vi "IVCurve Edit.vi"() -> ()   [LabVIEW 2019]
uses:
  Classes/Settings/Setting Database/Setting Database.lvclass
  Classes/Settings/Dot Settings/Dot Settings.lvclass
  Classes/Settings/Dot Settings/TypeDefs/IV Settings.ctl
  Classes/Settings/Dot Settings/Dot Settings.lvclass/Dot Settings.ctl
  <vilib>/JKI/JKI SMO/SMO/SMO.lvclass
panel:
  in  "Time":dbl caption="Time (s)"
  in  "Critical Points (V)":dbl[](array[numeric])
  out "Beta String":string
  in  "Pattern":T1(ring) caption="Enum"
  in  "Cycles":i32
  in  "Port":u32
  in  "End":dbl caption="End (V)"
  in  "Start":dbl caption="Start (V)"
  in  "Rate":dbl caption="Rate (V/s)"
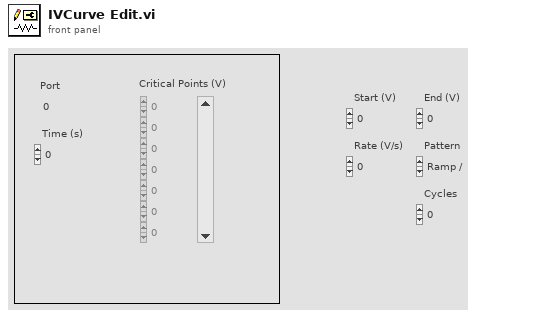
[diagram p1: front panel]
types:
  T1 = enum16{"Ramp /", "Ramp /\\", "Smooth Ramp _/", "Smooth Ramp _/\\_", "Frequency"}
  T2 = enum32{"Invalid", "Standard", "Closed", "Hidden", "Minimized", "Maximized"}
  T3 = enum32{"invalid app kind", "Development System", "Run Time System", "Student Edition", "Embedded LabVIEW", "Evaluation", "Custom"}
  T4 = typedef "Setting Database.lvclass/PublicEvents--Setting Database.NewActiveDot.ctl" = refnum<class "Dot Settings.lvclass">
  T5 = cluster{"Core":cluster{"Current VI Reference":refnum<vi>, "Close Panel on Exit?":bool}, "SettingDB":refnum<class "Setting Database.lvclass">, "Dot Settings":refnum<class "Dot Settings.lvclass">}
  T6 = typedef "Dot Settings.lvclass/IV Settings.ctl" = cluster{"Pattern":enum16{"Ramp /", "Ramp /\\", "Smooth Ramp _/", "Smooth Ramp _/\\_", "Frequency"}, "Cycles":i32, "Rate":dbl, "End":dbl, "Start":dbl, "Port":u32, "Time":dbl, "Points":dbl[]}
  T7 = cluster{"Current VI Reference":refnum<vi>, "Close Panel on Exit?":bool}
  T8 = typedef "Setting Database.lvclass/PublicEvents--Cluster.ctl" = cluster{"NewActivePath":refnum<user-event>, "PathsUpdated":refnum<user-event>, "RectanglesUpdated":refnum<user-event>, "NewActiveRectangle":refnum<user-event>, "NewActiveFunnel":refnum<user-event>, "FunnelsUpdated":refnum<user-event>, "NewActiveDot":refnum<user-event>, "DotsUpdated":refnum<user-event>}
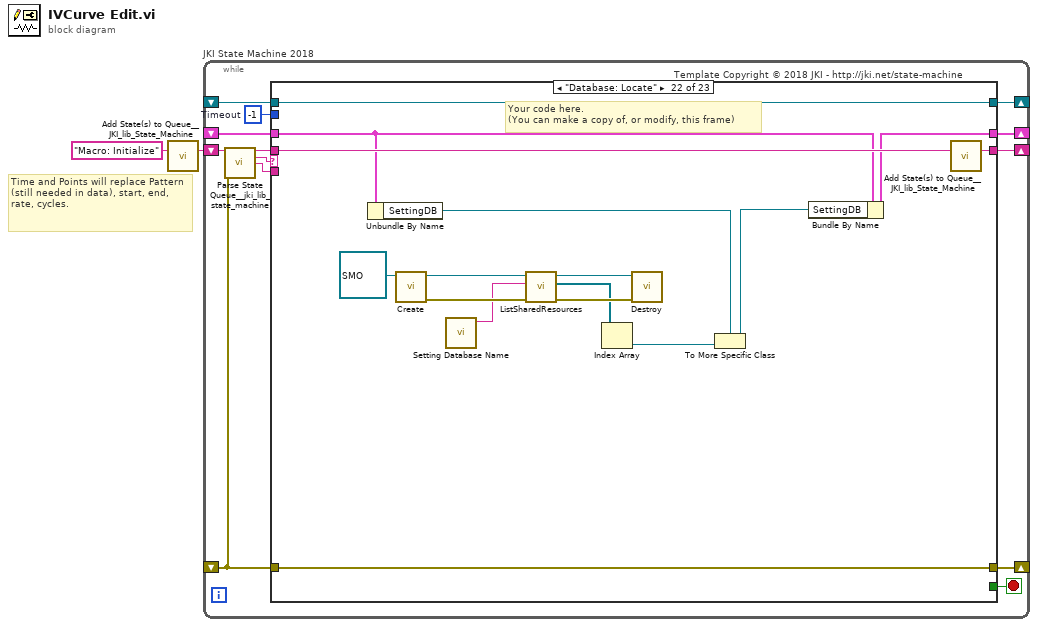
[diagram p0: block diagram]
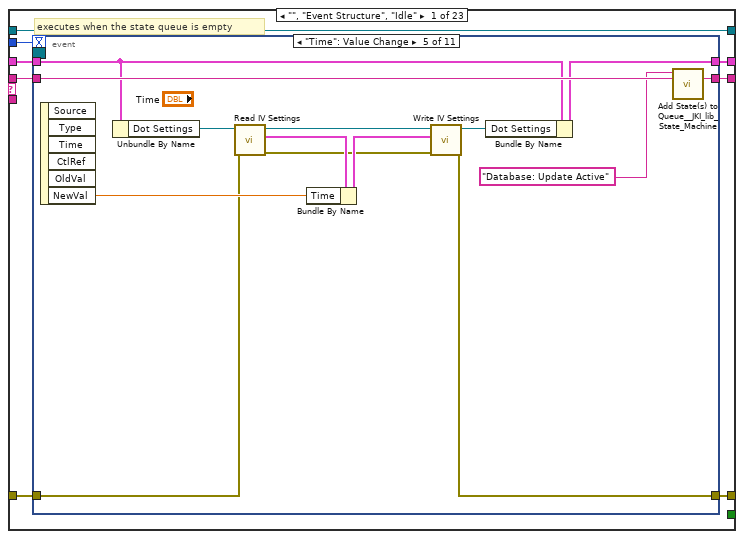
[diagram p2: hidden frame]
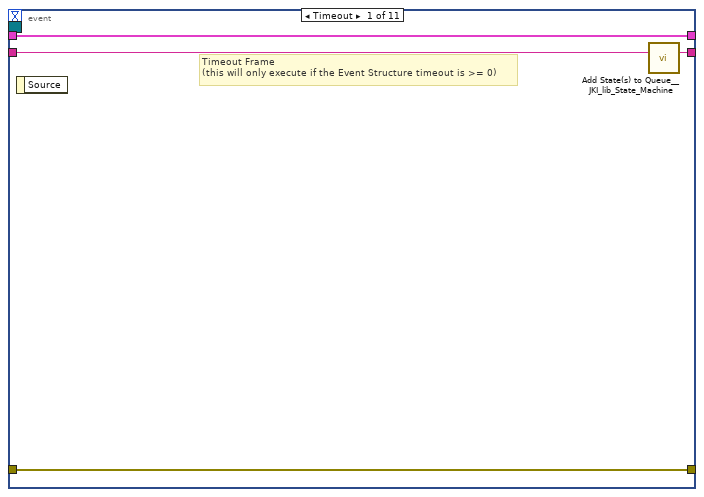
[diagram p3: hidden frame]
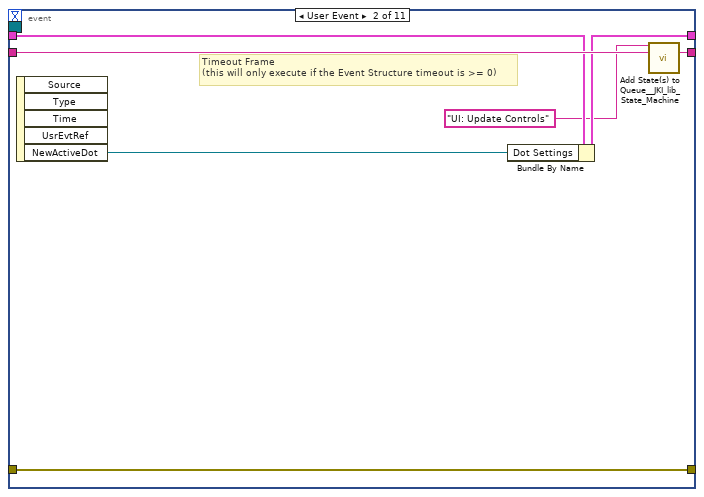
[diagram p4: hidden frame]
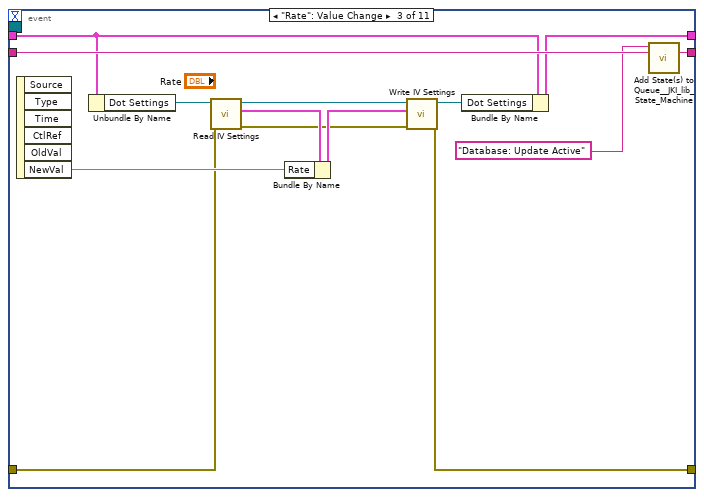
[diagram p5: hidden frame]
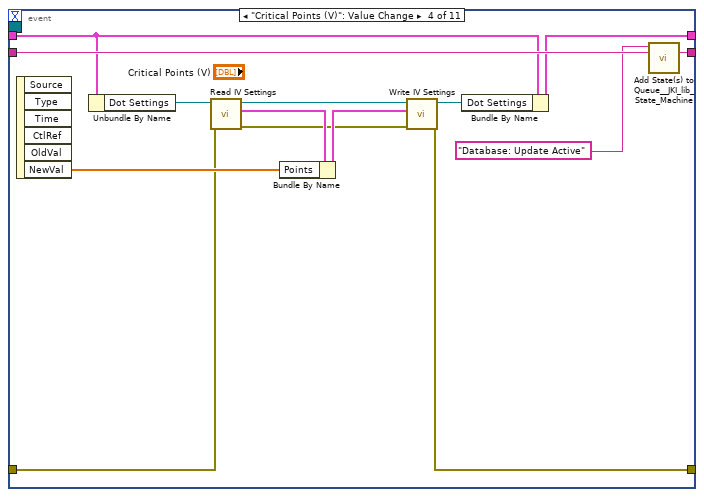
[diagram p6: hidden frame]
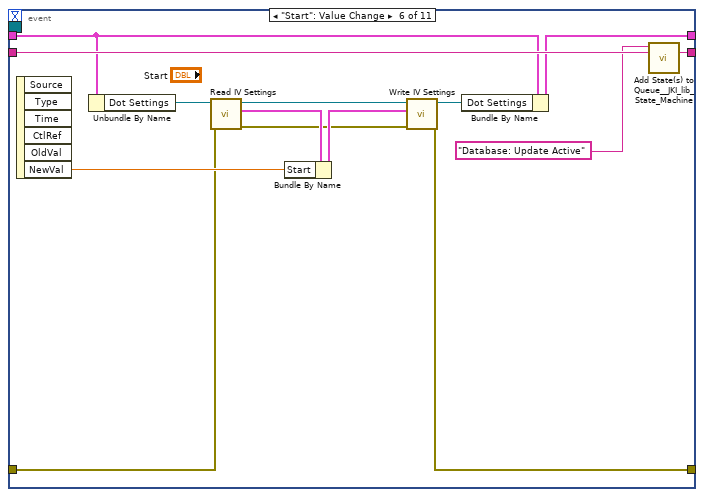
[diagram p7: hidden frame]
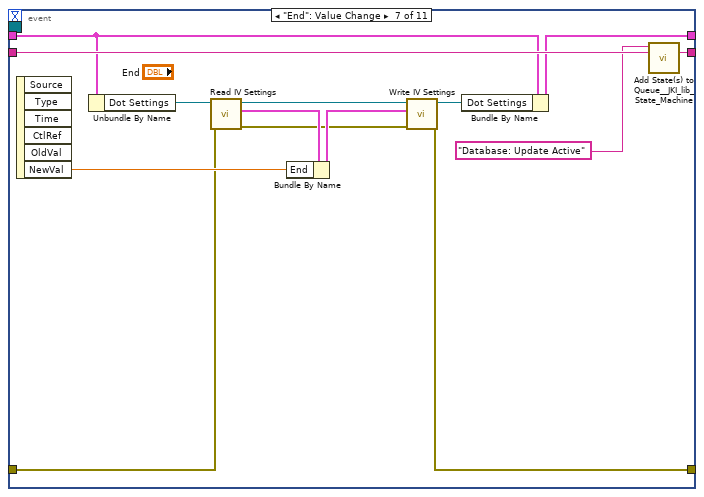
[diagram p8: hidden frame]
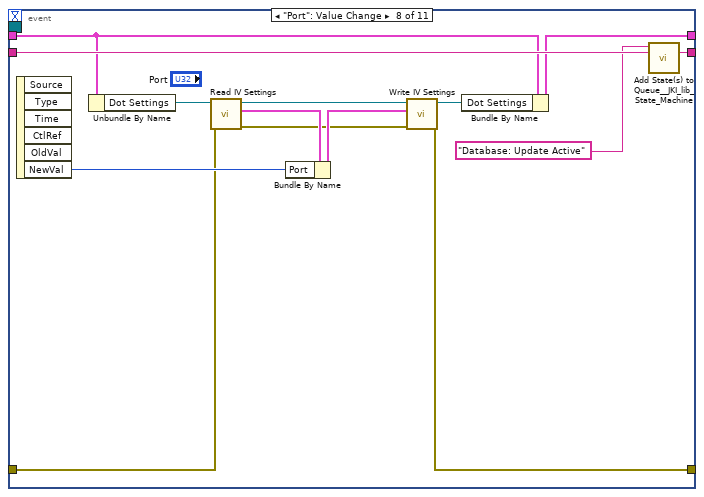
[diagram p9: hidden frame]
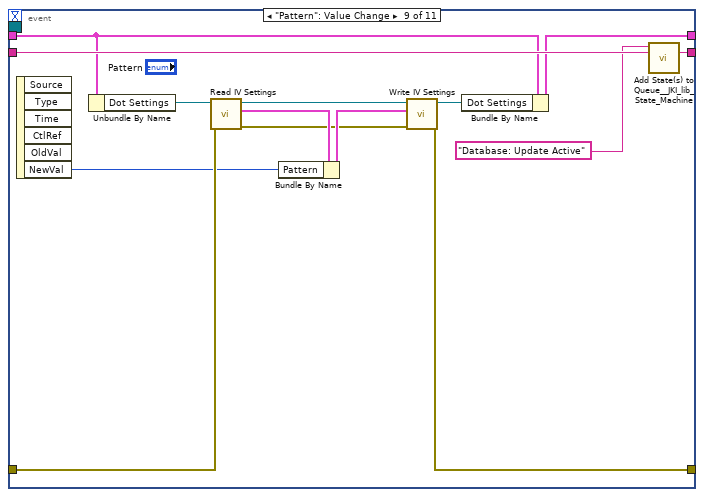
[diagram p10: hidden frame]
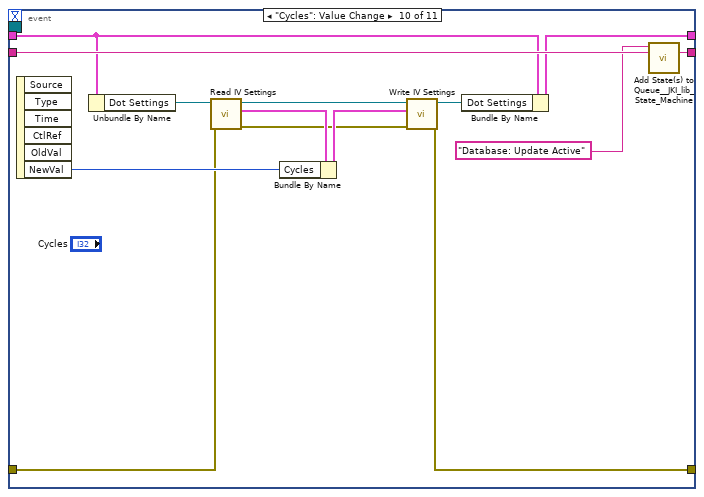
[diagram p11: hidden frame]
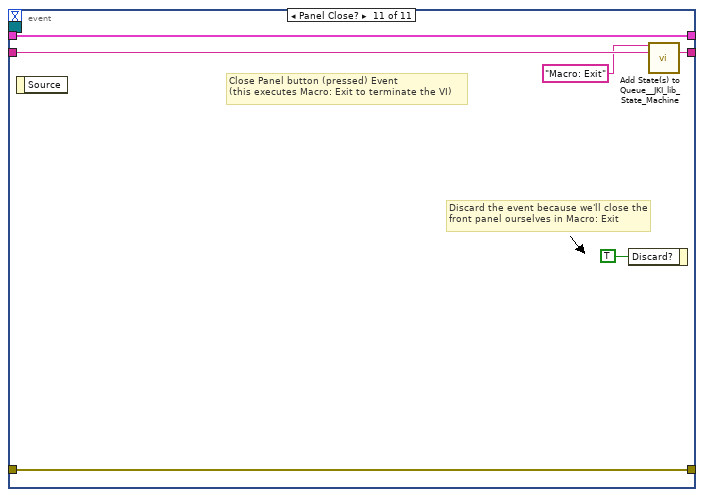
[diagram p12: hidden frame]
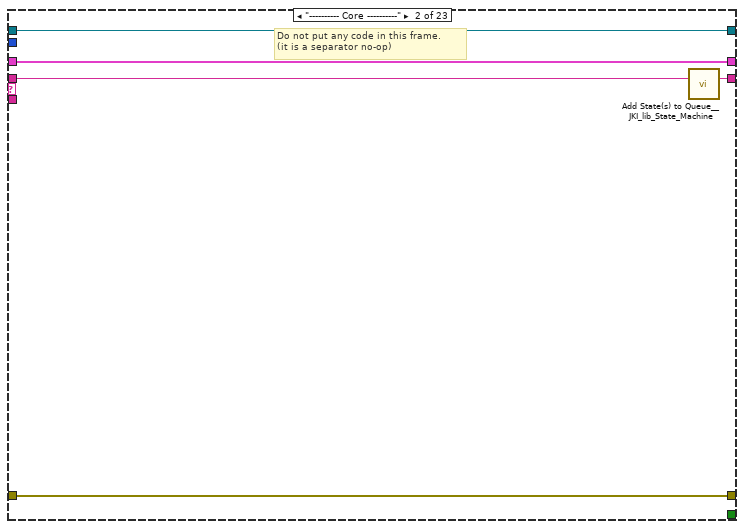
[diagram p13: hidden frame]
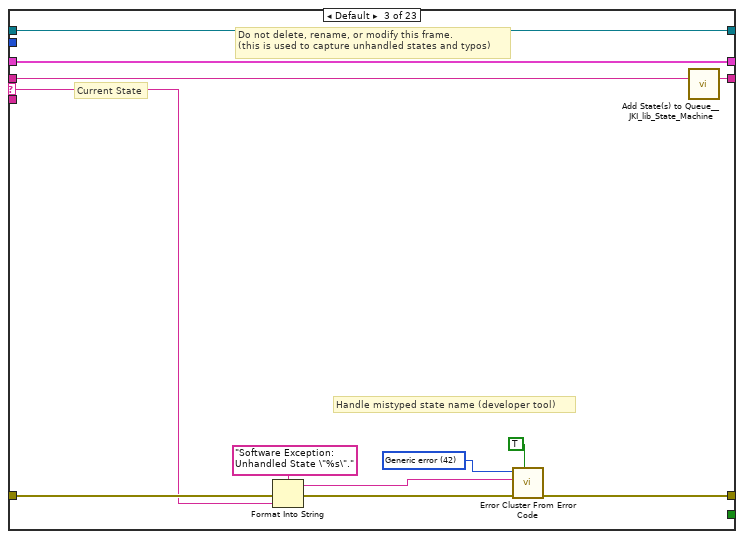
[diagram p14: hidden frame]
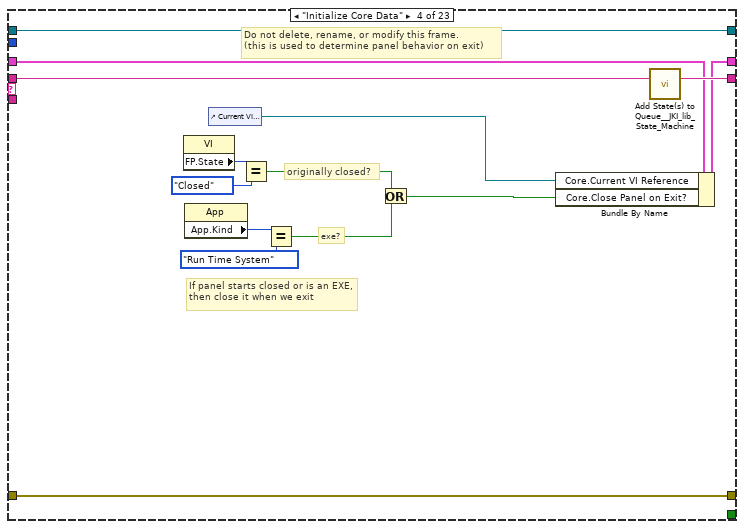
[diagram p15: hidden frame]
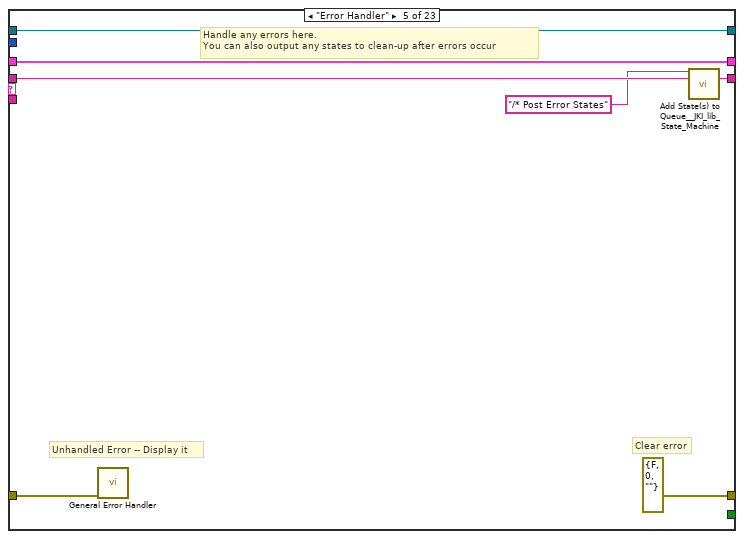
[diagram p16: hidden frame]
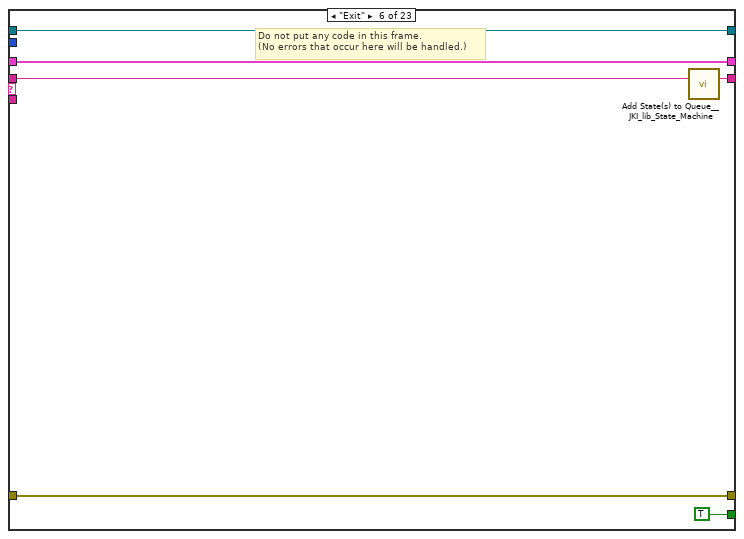
[diagram p17: hidden frame]
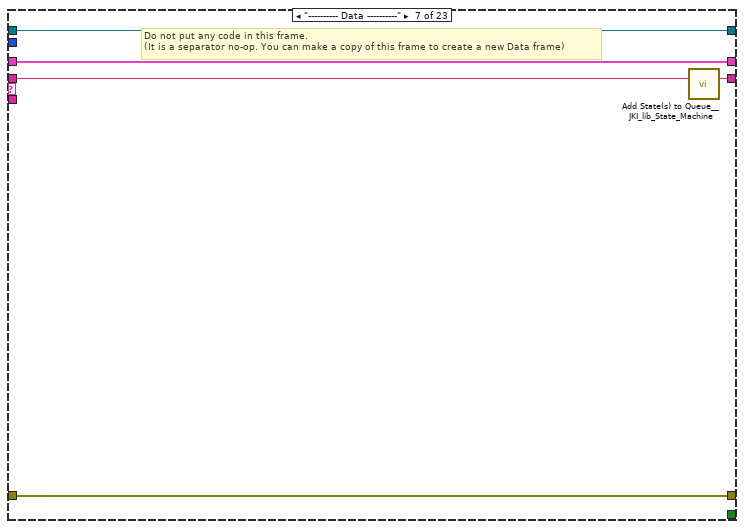
[diagram p18: hidden frame]
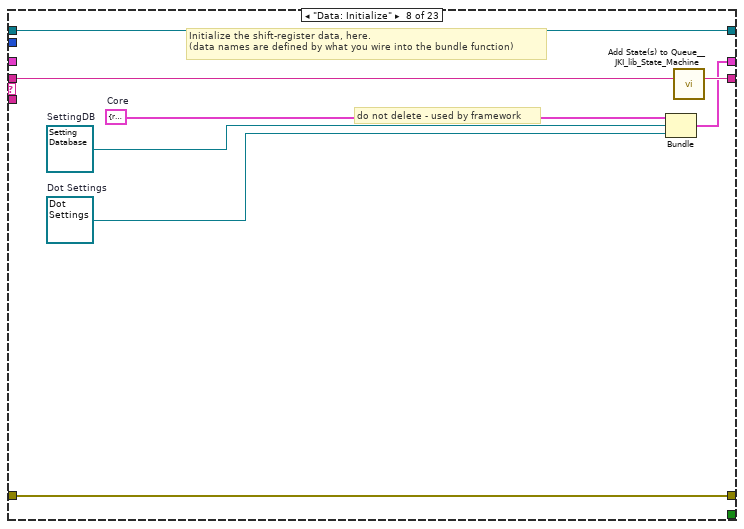
[diagram p19: hidden frame]
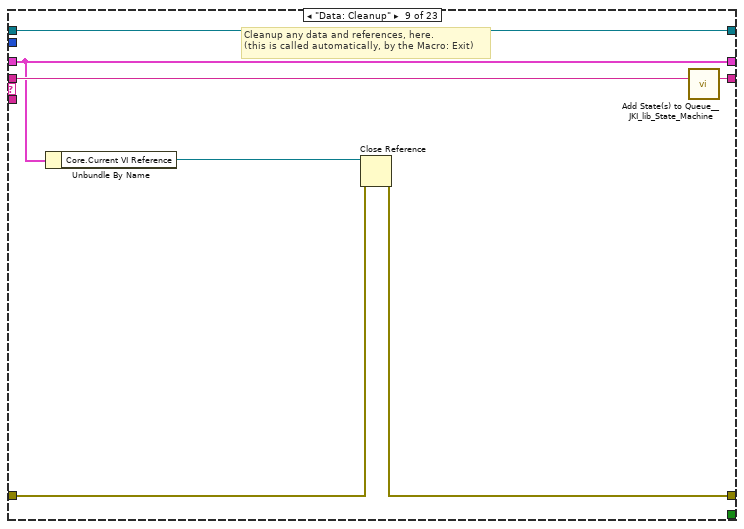
[diagram p20: hidden frame]
diagram:
  # "Time and Points will replace Pattern (still needed in data), start, end, rate, cycles."
  n1 = call <vilib>:"Add State(s) to Queue__JKI_lib_State_Machine.vi"("State(s) in (\"\")"="Macro: Initialize") -> ("States Out"=w2:string)  [unwired: 14 in]
  n2 = while "JKI State Machine 2018" {
    shift-right: [w8] -> _
    shift-left: _ -> [w7]
    shift-right: [w11] -> _
    shift-left: _ -> [w5]
    shift-right: [w10] -> _
    shift-left: w2 -> [w12]
    shift-right: [w4] -> _
    shift-left: _ -> [w3]
    stop <- w9 stop-if-true
    w6 = -1  # Timeout
    # "Template Copyright © 2018 JKI - http://jki.net/state-machine"
    n3 = call <vilib>:"Parse State Queue__jki_lib_state_machine.vi"("State Queue"=w12, "Error In (no error)"=w5) -> ("Remaining States"=w14:string, "Current State"=w15:string, "Arguments"=w13:string)  [unwired: 11 in]
    n4 = case shown="\"Database: Locate\"" w15 {
      selector: w15 -> [_ _ w159 _ _ _ _ _ _ _ _ _ _ _ _ _ _ _ _ _ _ _ _]
      tunnel: w14 -> [w23 w157 w163 w183 w190 w196 w201 w209 w216 w221 w229 w235 w240 w266 w281 w288 w300 w370 w376 w387 w392 w408 w418]
      tunnel: w13 -> [_ _ _ _ _ _ _ _ _ _ _ _ _ _ _ w283 w294 _ _ _ _ _ _]
      tunnel: w7 -> [w21 w154 w161 w176 w187 w194 w198 _ w211 w218 w225 w233 w237 w263 w279 w286 w296 w367 w373 w384 w389 w398 w410]
      tunnel: [w20 w155 w165 w180 errorcluster {"status"=FALSE, "code"=0, "source"=""} ("error out") w193 w199 w206 w212 w219 w226 w230 w238 w256 w278 w284 w297 w368 w374 w385 w390 w406 w414] -> w11
      tunnel: w5 -> [w19 w155 w164 w180 w186 w193 w199 w206 w213 w219 w223 w231 w238 w244 w278 w285 w298 w368 w374 w385 w390 w406 w413]
      tunnel: [w22 w156 w162 w182 w189 w195 w200 w208 w215 w220 w228 w234 w239 w265 w280 w287 w299 w369 w375 w386 w391 w407 w417] -> w10
      tunnel: [_ _ _ _ _ TRUE _ _ _ _ _ _ _ _ _ _ _ _ _ _ _ _ _] -> w9
      tunnel: [w18 w154 w161 w181 w187 w194 w198 w207 w211 w218 w225 w233 w237 w263 w279 w286 w296 w367 w373 w384 w389 w399 w412] -> w8
      tunnel: w6 -> [w17 _ _ _ _ _ _ _ _ _ _ _ _ _ _ _ _ _ _ _ _ _ _]
      tunnel: [w16 w153 w158 w170 w184 w191 w197 w202 w210 w217 w227 w232 w236 w264 w277 w282 w293 w366 w371 w377 w388 w394 w409] -> w4
      tunnel: w3 -> [w16 w153 w158 w170 w184 w191 w197 w202 w210 w217 _ w232 w236 w264 w277 w282 w293 w366 w371 w377 w388 w394 w409]
      frame "", "Event Structure", "Idle" {
        # "executes when the state queue is empty"
        n5 = event shown="[4] \"Time\": Value Change" {
          selector: w16 -> [_ _ _ _ _ _ _ _ _ _ _]
          dyn-events: _ -> [_ _ _ _ _ _ _ _ _ _ _]
          timeout: w17 -> [_ _ _ _ _ _ _ _ _ _ _]
          tunnel: w23 -> [w27 w34 w48 w62 w76 w90 w104 w118 w132 w146 w152]
          tunnel: [w26 w33 w47 w61 w75 w89 w103 w117 w131 w145 w151] -> w22
          tunnel: w21 -> [w24 w30 w45 w59 w73 w87 w101 w115 w129 w143 w149]
          tunnel: [w25 w32 w36 w50 w64 w78 w92 w106 w121 w134 w150] -> w20
          tunnel: w19 -> [w25 w32 w35 w49 w63 w77 w91 w105 w120 w133 w150]
          tunnel: [w24 w31 w46 w60 w74 w88 w102 w116 w130 w144 w149] -> w18
          event Timeout {
            # "Timeout Frame\n(this will only execute if the Event Structure timeout is >= 0)"
            n6 = event-data() -> ()  [unwired: 1 in, 1 out]
            n7 = call <vilib>:"Add State(s) to Queue__JKI_lib_State_Machine.vi"("State(s) in (\"\")"=w27) -> ("States Out"=w26:string)  [unwired: 14 in]
          }
          event User Event {
            # "Timeout Frame\n(this will only execute if the Event Structure timeout is >= 0)"
            n8 = event-data() -> ("NewActiveDot"=w29:T4)  [unwired: 1 in, 4 out]
            n9 = Bundle By Name(cluster=w30, "Dot Settings"=w29) -> (w31:T5)
            n10 = call <vilib>:"Add State(s) to Queue__JKI_lib_State_Machine.vi"("State(s) in Front (\"\")"="UI: Update Controls", "State(s) in (\"\")"=w34) -> ("States Out"=w33:string)  [unwired: 13 in]
          }
          event "Rate": Value Change {
            n11 = event-data() -> ("NewVal"=w41:dbl)  [unwired: 1 in, 5 out]
            n12 = Unbundle By Name(w45) -> ("Dot Settings"=w43:refnum<class "Dot Settings.lvclass">)
            n13 = call "Read IV Settings.vi"("error in (no error)"=w35, "Dot Settings in"=w43) -> ("error out"=w37:errorcluster, "IV Settings"=w42:T6, "Dot Settings out"=w40:refnum<class "Dot Settings.lvclass">)  [unwired: 7 in]
            n14 = Bundle By Name(cluster=w42, "Rate"=w41) -> (w38:T6)
            n15 = call "Write IV Settings.vi"("error in (no error)"=w37, "IV Settings"=w38, "Dot Settings in"=w40) -> ("error out"=w36:errorcluster, "Dot Settings out"=w39:refnum<class "Dot Settings.lvclass">)  [unwired: 7 in]
            n16 = Bundle By Name(cluster=w45, "Dot Settings"=w39) -> (w46:T5)
            n17 = call <vilib>:"Add State(s) to Queue__JKI_lib_State_Machine.vi"("State(s) in Front (\"\")"="Database: Update Active", "State(s) in (\"\")"=w48) -> ("States Out"=w47:string)  [unwired: 13 in]
          }
          event "Critical Points (V)": Value Change {
            n18 = event-data() -> ("NewVal"=w55:dbl[])  [unwired: 1 in, 5 out]
            n19 = Unbundle By Name(w59) -> ("Dot Settings"=w57:refnum<class "Dot Settings.lvclass">)
            n20 = call "Read IV Settings.vi"("error in (no error)"=w49, "Dot Settings in"=w57) -> ("error out"=w51:errorcluster, "IV Settings"=w56:T6, "Dot Settings out"=w54:refnum<class "Dot Settings.lvclass">)  [unwired: 7 in]
            n21 = Bundle By Name(cluster=w56, "Points"=w55) -> (w52:T6)
            n22 = call "Write IV Settings.vi"("error in (no error)"=w51, "IV Settings"=w52, "Dot Settings in"=w54) -> ("error out"=w50:errorcluster, "Dot Settings out"=w53:refnum<class "Dot Settings.lvclass">)  [unwired: 7 in]
            n23 = Bundle By Name(cluster=w59, "Dot Settings"=w53) -> (w60:T5)
            n24 = call <vilib>:"Add State(s) to Queue__JKI_lib_State_Machine.vi"("State(s) in Front (\"\")"="Database: Update Active", "State(s) in (\"\")"=w62) -> ("States Out"=w61:string)  [unwired: 13 in]
          }
          event "Time": Value Change {
            n25 = event-data() -> ("NewVal"=w69:dbl)  [unwired: 1 in, 5 out]
            n26 = Unbundle By Name(w73) -> ("Dot Settings"=w71:refnum<class "Dot Settings.lvclass">)
            n27 = call "Read IV Settings.vi"("error in (no error)"=w63, "Dot Settings in"=w71) -> ("error out"=w65:errorcluster, "IV Settings"=w70:T6, "Dot Settings out"=w68:refnum<class "Dot Settings.lvclass">)  [unwired: 7 in]
            n28 = Bundle By Name(cluster=w70, "Time"=w69) -> (w66:T6)
            n29 = call "Write IV Settings.vi"("error in (no error)"=w65, "IV Settings"=w66, "Dot Settings in"=w68) -> ("error out"=w64:errorcluster, "Dot Settings out"=w67:refnum<class "Dot Settings.lvclass">)  [unwired: 7 in]
            n30 = Bundle By Name(cluster=w73, "Dot Settings"=w67) -> (w74:T5)
            n31 = call <vilib>:"Add State(s) to Queue__JKI_lib_State_Machine.vi"("State(s) in Front (\"\")"="Database: Update Active", "State(s) in (\"\")"=w76) -> ("States Out"=w75:string)  [unwired: 13 in]
          }
          event "Start": Value Change {
            n32 = event-data() -> ("NewVal"=w83:dbl)  [unwired: 1 in, 5 out]
            n33 = Unbundle By Name(w87) -> ("Dot Settings"=w85:refnum<class "Dot Settings.lvclass">)
            n34 = call "Read IV Settings.vi"("error in (no error)"=w77, "Dot Settings in"=w85) -> ("error out"=w79:errorcluster, "IV Settings"=w84:T6, "Dot Settings out"=w82:refnum<class "Dot Settings.lvclass">)  [unwired: 7 in]
            n35 = Bundle By Name(cluster=w84, "Start"=w83) -> (w80:T6)
            n36 = call "Write IV Settings.vi"("error in (no error)"=w79, "IV Settings"=w80, "Dot Settings in"=w82) -> ("error out"=w78:errorcluster, "Dot Settings out"=w81:refnum<class "Dot Settings.lvclass">)  [unwired: 7 in]
            n37 = Bundle By Name(cluster=w87, "Dot Settings"=w81) -> (w88:T5)
            n38 = call <vilib>:"Add State(s) to Queue__JKI_lib_State_Machine.vi"("State(s) in Front (\"\")"="Database: Update Active", "State(s) in (\"\")"=w90) -> ("States Out"=w89:string)  [unwired: 13 in]
          }
          event "End": Value Change {
            n39 = event-data() -> ("NewVal"=w97:dbl)  [unwired: 1 in, 5 out]
            n40 = Unbundle By Name(w101) -> ("Dot Settings"=w99:refnum<class "Dot Settings.lvclass">)
            n41 = call "Read IV Settings.vi"("error in (no error)"=w91, "Dot Settings in"=w99) -> ("error out"=w93:errorcluster, "IV Settings"=w98:T6, "Dot Settings out"=w96:refnum<class "Dot Settings.lvclass">)  [unwired: 7 in]
            n42 = Bundle By Name(cluster=w98, "End"=w97) -> (w94:T6)
            n43 = call "Write IV Settings.vi"("error in (no error)"=w93, "IV Settings"=w94, "Dot Settings in"=w96) -> ("error out"=w92:errorcluster, "Dot Settings out"=w95:refnum<class "Dot Settings.lvclass">)  [unwired: 7 in]
            n44 = Bundle By Name(cluster=w101, "Dot Settings"=w95) -> (w102:T5)
            n45 = call <vilib>:"Add State(s) to Queue__JKI_lib_State_Machine.vi"("State(s) in Front (\"\")"="Database: Update Active", "State(s) in (\"\")"=w104) -> ("States Out"=w103:string)  [unwired: 13 in]
          }
          event "Port": Value Change {
            n46 = event-data() -> ("NewVal"=w111:u32)  [unwired: 1 in, 5 out]
            n47 = Unbundle By Name(w115) -> ("Dot Settings"=w113:refnum<class "Dot Settings.lvclass">)
            n48 = call "Read IV Settings.vi"("error in (no error)"=w105, "Dot Settings in"=w113) -> ("error out"=w107:errorcluster, "IV Settings"=w112:T6, "Dot Settings out"=w110:refnum<class "Dot Settings.lvclass">)  [unwired: 7 in]
            n49 = Bundle By Name(cluster=w112, "Port"=w111) -> (w108:T6)
            n50 = call "Write IV Settings.vi"("error in (no error)"=w107, "IV Settings"=w108, "Dot Settings in"=w110) -> ("error out"=w106:errorcluster, "Dot Settings out"=w109:refnum<class "Dot Settings.lvclass">)  [unwired: 7 in]
            n51 = Bundle By Name(cluster=w115, "Dot Settings"=w109) -> (w116:T5)
            n52 = call <vilib>:"Add State(s) to Queue__JKI_lib_State_Machine.vi"("State(s) in Front (\"\")"="Database: Update Active", "State(s) in (\"\")"=w118) -> ("States Out"=w117:string)  [unwired: 13 in]
          }
          event "Pattern": Value Change {
            n53 = event-data() -> ("NewVal"=w119:T1)  [unwired: 1 in, 5 out]
            n54 = Unbundle By Name(w129) -> ("Dot Settings"=w127:refnum<class "Dot Settings.lvclass">)
            n55 = call "Read IV Settings.vi"("error in (no error)"=w120, "Dot Settings in"=w127) -> ("error out"=w122:errorcluster, "IV Settings"=w126:T6, "Dot Settings out"=w125:refnum<class "Dot Settings.lvclass">)  [unwired: 7 in]
            n56 = Bundle By Name(cluster=w126, "Pattern"=w119) -> (w123:T6)
            n57 = call "Write IV Settings.vi"("error in (no error)"=w122, "IV Settings"=w123, "Dot Settings in"=w125) -> ("error out"=w121:errorcluster, "Dot Settings out"=w124:refnum<class "Dot Settings.lvclass">)  [unwired: 7 in]
            n58 = Bundle By Name(cluster=w129, "Dot Settings"=w124) -> (w130:T5)
            n59 = call <vilib>:"Add State(s) to Queue__JKI_lib_State_Machine.vi"("State(s) in Front (\"\")"="Database: Update Active", "State(s) in (\"\")"=w132) -> ("States Out"=w131:string)  [unwired: 13 in]
          }
          event "Cycles": Value Change {
            n60 = event-data() -> ("NewVal"=w139:i32)  [unwired: 1 in, 5 out]
            n61 = Unbundle By Name(w143) -> ("Dot Settings"=w141:refnum<class "Dot Settings.lvclass">)
            n62 = call "Read IV Settings.vi"("error in (no error)"=w133, "Dot Settings in"=w141) -> ("error out"=w135:errorcluster, "IV Settings"=w140:T6, "Dot Settings out"=w138:refnum<class "Dot Settings.lvclass">)  [unwired: 7 in]
            n63 = Bundle By Name(cluster=w140, "Cycles"=w139) -> (w136:T6)
            n64 = call "Write IV Settings.vi"("error in (no error)"=w135, "IV Settings"=w136, "Dot Settings in"=w138) -> ("error out"=w134:errorcluster, "Dot Settings out"=w137:refnum<class "Dot Settings.lvclass">)  [unwired: 7 in]
            n65 = Bundle By Name(cluster=w143, "Dot Settings"=w137) -> (w144:T5)
            n66 = call <vilib>:"Add State(s) to Queue__JKI_lib_State_Machine.vi"("State(s) in Front (\"\")"="Database: Update Active", "State(s) in (\"\")"=w146) -> ("States Out"=w145:string)  [unwired: 13 in]
          }
          event Panel Close? {
            # "Discard the event because we'll close the front panel ourselves in Macro: Exit"
            # "Close Panel button (pressed) Event\n(this executes Macro: Exit to terminate the VI)"
            n67 = event-data() -> ()  [unwired: 1 in, 1 out]
            n68 = event-data("Discard?"=TRUE) -> ()  [unwired: 1 in, 1 out]
            n69 = call <vilib>:"Add State(s) to Queue__JKI_lib_State_Machine.vi"("State(s) in Front (\"\")"="Macro: Exit", "State(s) in (\"\")"=w152) -> ("States Out"=w151:string)  [unwired: 13 in]
          }
        }
      }
      frame "---------- Core ----------" {
        # "Do not put any code in this frame.\n(it is a separator no-op)"
        n70 = call <vilib>:"Add State(s) to Queue__JKI_lib_State_Machine.vi"("State(s) in (\"\")"=w157) -> ("States Out"=w156:string)  [unwired: 14 in]
      }
      frame Default {
        w168 = 42 items=["No error", "Argument error", "Memory is full", "Out of zone", "End of file", "File already open", "Generic file I/O error", "File not found", "File permission error", "Disk is full", "Duplicate path", "Too many files open", "System feature not enabled", "Resource file not found", "Cannot add resource", "Resource not found", "Image not found", "Image memory error", "Pen does not exist", "Config type invalid", "Config token not found", "Config parse error", "Config memory error", "Bad external code format", "Bad external code offset", "External code not present", "Null window", "Destroy window error", "Null menu", "Print aborted", "Bad print record", "Print driver error", "Windows error during printing", "Memory error during printing", "Print dialog error", "Generic print error", "Invalid device refnum", "Device not found", "Device parameter error", "Device unit error", "Cannot open device", "Device call aborted", "Generic error", "Cancelled by user", "Object ID too low", "Object ID too high", "Object not in heap", "Unknown heap", "Unknown object (invalid DefProc)", "Unknown object (DefProc not in table)", "Message out of range", "Invalid (null) method", "Unknown message", "Manager call not supported", "Bad address", "Network operation in progress", "Network operation timed out", "Connection is busy", "Network attribute not supported", "Network error", "Address in use", "System out of memory", "Connection aborted", "Connection refused", "Not connected", "Already connected", "Connection closed", "Initialization error (interapplication manager)", "Bad occurrence", "Wait on unbound occurrence handler", "Occurrence queue overflow", "Datalog type conflict", "Unused", "Unrecognized type (interapplication manager)", "Memory corrupt", "Failed to make temporary DLL", "Old CIN version", "Drag socket not found", "Failed to load drop-object", "Failed to register OLE object", "Failed to release OLE object", "Format specifier type mismatch", "Unknown format specifier", "Too few format specifiers", "Too many format specifiers", "Scan failed", "Newer CIN version", "Error converting to variant", "Runtime menu error", "Password tampered", "Variant attribute not found", "Incompatible variant data type", "Event data is not available", "Event Store is not present", "Occurrence is not found", "Event Queue is not created", "Event info is not available", "Refnum passed is NULL", "Error retrieving Class GUID", "Error retrieving CoClass GUID", "Error retrieving TypeLib GUID.", "Bad built application magic bytes.", "Specific driver is different from the specific driver associated with the Logical Name.", "There is no session opened to the class driver.", "Max Error", "MAX - Error with config objects", "MAX - Error loading configuration", "MAX - Group not supported"]
        # "Current State"
        # "Do not delete, rename, or modify this frame.\n(this is used to capture unhandled states and typos)"
        # "Handle mistyped state name (developer tool)"
        n71 = Format Into String(format string="Software Exception: Unhandled State \"%s\"." ("message"), error in=w164, w159) -> (resulting string=w167:string, error out=w166:errorcluster)  [unwired: 1 in]
        n72 = call <vilib>:"Error Cluster From Error Code.vi"("show call chain? (False)"=TRUE, "error in (no error)"=w166, "error message (\"\")"=w167, "error code (0)"=w168) -> ("error out"=w165:errorcluster)  [unwired: 5 in]
        n73 = call <vilib>:"Add State(s) to Queue__JKI_lib_State_Machine.vi"("State(s) in (\"\")"=w163) -> ("States Out"=w162:string)  [unwired: 14 in]
      }
      frame "Initialize Core Data" {
        # "Do not delete, rename, or modify this frame.\n(this is used to determine panel behavior on exit)"
        # "originally closed?"
        # "exe?"
        # "If panel starts closed or is an EXE, then close it when we exit"
        n74 = property class="VI"() -> ("FP.State"=w173:T2)  [unwired: 2 in, 2 out]
        n75 = property class="App"() -> ("App.Kind"=w179:T3)  [unwired: 2 in, 2 out]
        n76 = control-ref of="Current VI Reference"() -> (w174:refnum<vi>)
        n77 = Equal?(x=w173, y=T2."Closed" ("Front Panel Window:State")) -> (x = y?=w171:bool)
        n78 = Equal?(x=w179, y=T3."Run Time System" ("Application:Kind")) -> (x = y?=w177:bool)
        n79 = Or(x=w171, y=w177) -> (x .or. y?=w175:bool)
        n80 = Bundle By Name(cluster=w176, "Core.Current VI Reference"=w174, "Core.Close Panel on Exit?"=w175) -> (w181:T5)
        n81 = call <vilib>:"Add State(s) to Queue__JKI_lib_State_Machine.vi"("State(s) in (\"\")"=w183) -> ("States Out"=w182:string)  [unwired: 14 in]
      }
      frame "Error Handler" {
        # "Unhandled Error -- Display it"
        # "Handle any errors here.\nYou can also output any states to clean-up after errors occur"
        # "Clear error"
        n82 = call <vilib>:"General Error Handler.vi"("error in (no error)"=w186) -> ()  [unwired: 10 in, 5 out]
        n83 = call <vilib>:"Add State(s) to Queue__JKI_lib_State_Machine.vi"("State(s) in Front (\"\")"="/* Post Error States", "State(s) in (\"\")"=w190) -> ("States Out"=w189:string)  [unwired: 13 in]
      }
      frame "Exit" {
        # "Do not put any code in this frame.\n(No errors that occur here will be handled.)"
        n84 = call <vilib>:"Add State(s) to Queue__JKI_lib_State_Machine.vi"("State(s) in (\"\")"=w196) -> ("States Out"=w195:string)  [unwired: 14 in]
      }
      frame "---------- Data ----------" {
        # "Do not put any code in this frame.\n(It is a separator no-op. You can make a copy of this frame to create a new Data frame)"
        n85 = call <vilib>:"Add State(s) to Queue__JKI_lib_State_Machine.vi"("State(s) in (\"\")"=w201) -> ("States Out"=w200:string)  [unwired: 14 in]
      }
      frame "Data: Initialize" {
        w203 = refnum<class "Dot Settings.lvclass"> refnum  # Dot Settings
        w204 = refnum<class "Setting Database.lvclass"> refnum  # SettingDB
        w205 = T7 {"Current VI Reference"=refnum, "Close Panel on Exit?"=FALSE}  # Core
        # "do not delete - used by framework"
        # "Initialize the shift-register data, here.\n(data names are defined by what you wire into the bundle function)"
        n86 = Bundle("Core"=w205, "SettingDB"=w204, "Dot Settings"=w203) -> (w207:T5)  [unwired: 1 in]
        n87 = call <vilib>:"Add State(s) to Queue__JKI_lib_State_Machine.vi"("State(s) in (\"\")"=w209) -> ("States Out"=w208:string)  [unwired: 14 in]
      }
      frame "Data: Cleanup" {
        # "Cleanup any data and references, here.\n(this is called automatically, by the Macro: Exit)"
        n88 = Unbundle By Name(w211) -> ("Core.Current VI Reference"=w214:refnum<vi>)
        n89 = Close Reference(reference=w214, error in (no error)=w213) -> (error out=w212:errorcluster)
        n90 = call <vilib>:"Add State(s) to Queue__JKI_lib_State_Machine.vi"("State(s) in (\"\")"=w216) -> ("States Out"=w215:string)  [unwired: 14 in]
      }
      frame "---------- Events ----------" {
        # "Do not put any code in this frame.\n(It is a separator no-op. You can make a copy of this frame to create a new UI frame)"
        n91 = call <vilib>:"Add State(s) to Queue__JKI_lib_State_Machine.vi"("State(s) in (\"\")"=w221) -> ("States Out"=w220:string)  [unwired: 14 in]
      }
      frame "Events: Register" {
        # "Do not put any code in this frame.\n(It is a separator no-op. You can make a copy of this frame to create a new UI frame)"
        n92 = Unbundle By Name(w225) -> ("SettingDB"=w224:refnum<class "Setting Database.lvclass">)
        n93 = call "Setting Database.GetPublicEvents.vi"("Setting Database"=w224) -> ("Public Events"=w222:T8)  [unwired: 8 in, 2 out]
        n94 = register-events(error in=w223, w222) -> (reference out=w227:refnum<event-registration>, error out=w226:errorcluster)  [unwired: 1 in]
        n95 = call <vilib>:"Add State(s) to Queue__JKI_lib_State_Machine.vi"("State(s) in (\"\")"=w229) -> ("States Out"=w228:string)  [unwired: 14 in]
      }
      frame "Events: Unregister" {
        # "Do not put any code in this frame.\n(It is a separator no-op. You can make a copy of this frame to create a new UI frame)"
        n96 = Unregister For Events(event registration refnum=w232, error in=w231) -> (error out=w230:errorcluster)
        n97 = call <vilib>:"Add State(s) to Queue__JKI_lib_State_Machine.vi"("State(s) in (\"\")"=w235) -> ("States Out"=w234:string)  [unwired: 14 in]
      }
      frame "---------- UI ----------" {
        # "Do not put any code in this frame.\n(It is a separator no-op. You can make a copy of this frame to create a new UI frame)"
        n98 = call <vilib>:"Add State(s) to Queue__JKI_lib_State_Machine.vi"("State(s) in (\"\")"=w240) -> ("States Out"=w239:string)  [unwired: 14 in]
      }
      frame "UI: Update Controls" {
        w243 = T6 {"Pattern"=enum."Ramp /", "Cycles"=1, "Rate"=1.0, "End"=-1.0, "Start"=1.0, "Port"=42069, "Time"=0.0, "Points"=[]} ("IV Settings")
        # "Do not put any code in this frame.\n(It is a separator no-op. You can make a copy of this frame to create a new UI frame)"
        n99 = Unbundle By Name(w263) -> ("Dot Settings"=w254:refnum<class "Dot Settings.lvclass">)
        n100 = call "Read Settings.vi"("error in (no error)"=w244, "Dot Settings in"=w254) -> ("error out"=w248:errorcluster, "Settings"=w253:variant, "Dot Settings out"=w251:refnum<class "Dot Settings.lvclass">)  [unwired: 7 in]
        n101 = call <userlib>:"Get Data Name__ogtk.vi"("error in (no error)"=w248, "Data"=w243) -> ("error out"=w247:errorcluster, "Data Name"=w252:string)  [unwired: 7 in, 1 out]
        n102 = Get Variant Attribute(Variant=w253, name=w252, error in=w247) -> (found=w249:bool, error out=w246:errorcluster)  [unwired: 1 in, 2 out]
        n103 = case shown="False" w249 {
          tunnel: w251 -> [w271 w273]
          tunnel: [w270 w273] -> w250
          tunnel: w246 -> [w269 w272]
          tunnel: [w268 w272] -> w245
          tunnel: w243 -> [w267 _]
          frame False {
            n104 = call "Write IV Settings.vi"("error in (no error)"=w269, "IV Settings"=w267, "Dot Settings in"=w271) -> ("error out"=w268:errorcluster, "Dot Settings out"=w270:refnum<class "Dot Settings.lvclass">)  [unwired: 7 in]
          }
          frame True {
          }
        }
        n105 = call "Read IV Settings.vi"("error in (no error)"=w245, "Dot Settings in"=w250) -> ("error out"=w256:errorcluster, "IV Settings"=w262:T6)  [unwired: 7 in, 1 out]
        n106 = Unbundle By Name(w262) -> ("Start"=w261:dbl, "Pattern"=w255:T1, "End"=w257:dbl, "Cycles"=w258:i32, "Rate"=w259:dbl, "Port"=w260:u32, "Time"=w242:dbl, "Points"=w241:dbl[])
        n107 = local write "Critical Points (V)"(w241) -> ()
        n108 = local write "Time"(w242) -> ()
        n109 = local write "Pattern"(w255) -> ()
        n110 = local write "Start"(w261) -> ()
        n111 = local write "End"(w257) -> ()
        n112 = local write "Cycles"(w258) -> ()
        n113 = local write "Rate"(w259) -> ()
        n114 = local write "Port"(w260) -> ()
        n115 = call <vilib>:"Add State(s) to Queue__JKI_lib_State_Machine.vi"("State(s) in (\"\")"=w266) -> ("States Out"=w265:string)  [unwired: 14 in]
      }
      frame "UI: Initialize" {
        # "Initialize the User Interface, here.\n(this is called automatically, by the Macro: Init)"
        n116 = call <userlib>:"MGI Get Executable Version.vi"() -> ("Version"=w276:string)  [unwired: 7 in]
        n117 = Concatenate Strings("Beta in v", w276) -> (→"Beta String":string)
        n118 = call <vilib>:"Add State(s) to Queue__JKI_lib_State_Machine.vi"("State(s) in (\"\")"=w281) -> ("States Out"=w280:string)  [unwired: 14 in]
      }
      frame "UI: Cursor Set" {
        # "Argument"
        # "Set and Unset Cursor Busy.\n(Usage: \"UI: Cursor Set >> Busy|Idle\")"
        n119 = case shown="\"Idle\", Default" w283 {
          tunnel: w285 -> [w290 w292]
          tunnel: [w289 w291] -> w284
          frame "Idle", Default {
            n120 = call <vilib>:"Unset Busy.vi"("error in (no error)"=w290) -> ("error out"=w289:errorcluster)  [unwired: 10 in]
          }
          frame "Busy" {
            n121 = call <vilib>:"Set Busy.vi"("error in (no error)"=w292) -> ("error out"=w291:errorcluster)  [unwired: 9 in, 1 out]
          }
        }
        n122 = call <vilib>:"Add State(s) to Queue__JKI_lib_State_Machine.vi"("State(s) in (\"\")"=w288) -> ("States Out"=w287:string)  [unwired: 14 in]
      }
      frame "UI: Front Panel State" {
        # "Argument"
        # "Set Front Panel Open or Closed\n(Usage: \"UI: Front Panel State >> Open|Close\")"
        n123 = Unbundle By Name(w296) -> ("Core.Current VI Reference"=w295:refnum<vi>)
        n124 = case shown="\"Close\", \"Closed\"" w294 {
          tunnel: w298 -> [w306 w321 w332 w345 w358]
          tunnel: [w308 w322 w334 w347 w360] -> w297
          tunnel: w295 -> [w307 w319 w333 w346 w359]
          frame "Open", "Standard", Default {
            w301 = T2."Standard" ("State")
            n125 = property class="VI"(reference=w307, error in=w306) -> (reference out=w304:refnum<vi>, error out=w305:errorcluster, "FP.State"=w303:T2)
            n126 = Not Equal?(x=w303, y=w301) -> (x != y?=w302:bool)
            n127 = case shown="True" w302 {
              tunnel: [w312 w314] -> w308
              tunnel: w305 -> [w311 w314]
              tunnel: w304 -> [w310 _]
              tunnel: w301 -> [w309 _]
              frame True {
                n128 = invoke class="VI" method="FP.Open"(reference=w310, error in=w311, "Activate"=TRUE, "State"=w309) -> (error out=w312:errorcluster)  [unwired: 1 in, 4 out]
              }
              frame False {
              }
            }
          }
          frame "Close", "Closed" {
            n129 = property class="VI"(reference=w319, error in=w321) -> (reference out=w318:refnum<vi>, error out=w320:errorcluster, "FP.State"=w316:T2)
            n130 = Not Equal?(x=w316, y=T2."Closed" ("Front Panel Window:State")) -> (x != y?=w315:bool)
            n131 = case shown="True" w315 {
              tunnel: [w323 w326] -> w322
              tunnel: w320 -> [w323 w325]
              tunnel: w318 -> [_ w324]
              frame False {
              }
              frame True {
                n132 = invoke class="VI" method="FP.Close"(reference=w324, error in=w325) -> (error out=w326:errorcluster)  [unwired: 1 in, 2 out]
              }
            }
          }
          frame "Hidden", "Hide" {
            w327 = T2."Hidden" ("State")
            n133 = property class="VI"(reference=w333, error in=w332) -> (reference out=w330:refnum<vi>, error out=w331:errorcluster, "FP.State"=w329:T2)
            n134 = Not Equal?(x=w329, y=w327) -> (x != y?=w328:bool)
            n135 = case shown="True" w328 {
              tunnel: [w338 w339] -> w334
              tunnel: w331 -> [w337 w339]
              tunnel: w330 -> [w336 _]
              tunnel: w327 -> [w335 _]
              frame True {
                n136 = invoke class="VI" method="FP.Open"(reference=w336, error in=w337, "State"=w335) -> (error out=w338:errorcluster)  [unwired: 2 in, 4 out]
              }
              frame False {
              }
            }
          }
          frame "Minimize", "Minimized" {
            w340 = T2."Minimized" ("State")
            n137 = property class="VI"(reference=w346, error in=w345) -> (reference out=w343:refnum<vi>, error out=w344:errorcluster, "FP.State"=w342:T2)
            n138 = Not Equal?(x=w342, y=w340) -> (x != y?=w341:bool)
            n139 = case shown="True" w341 {
              tunnel: [w351 w352] -> w347
              tunnel: w344 -> [w350 w352]
              tunnel: w343 -> [w349 _]
              tunnel: w340 -> [w348 _]
              frame True {
                n140 = invoke class="VI" method="FP.Open"(reference=w349, error in=w350, "State"=w348) -> (error out=w351:errorcluster)  [unwired: 2 in, 4 out]
              }
              frame False {
              }
            }
          }
          frame "Maximize", "Maximized" {
            w353 = T2."Maximized" ("State")
            n141 = property class="VI"(reference=w359, error in=w358) -> (reference out=w356:refnum<vi>, error out=w357:errorcluster, "FP.State"=w355:T2)
            n142 = Not Equal?(x=w355, y=w353) -> (x != y?=w354:bool)
            n143 = case shown="True" w354 {
              tunnel: [w364 w365] -> w360
              tunnel: w357 -> [w363 w365]
              tunnel: w356 -> [w362 _]
              tunnel: w353 -> [w361 _]
              frame True {
                n144 = invoke class="VI" method="FP.Open"(reference=w362, error in=w363, "State"=w361) -> (error out=w364:errorcluster)  [unwired: 2 in, 4 out]
              }
              frame False {
              }
            }
          }
        }
        n145 = call <vilib>:"Add State(s) to Queue__JKI_lib_State_Machine.vi"("State(s) in (\"\")"=w300) -> ("States Out"=w299:string)  [unwired: 14 in]
      }
      frame "---------- Macro ----------" {
        # "Do not put any code in this frame.\n(It is a separator no-op. You can make a copy of this frame to create a new Macro frame)"
        n146 = call <vilib>:"Add State(s) to Queue__JKI_lib_State_Machine.vi"("State(s) in (\"\")"=w370) -> ("States Out"=w369:string)  [unwired: 14 in]
      }
      frame "Macro: Initialize" {
        # "Initialization Macro\n(This is called once, when the VI starts)"
        n147 = call <vilib>:"Add State(s) to Queue__JKI_lib_State_Machine.vi"("State(s) in Front (\"\")"="Data: Initialize\nInitialize Core Data\nDatabase: Locate\nEvents: Register\nUI: Initialize\nUI: Update Controls\nUI: Front Panel State >> Closed", "State(s) in (\"\")"=w376) -> ("States Out"=w375:string)  [unwired: 13 in]
      }
      frame "Macro: Exit" {
        # "Exit Macro\n(This is called once, when the VI exits)"
        n148 = Unbundle By Name(w384) -> ("Core.Close Panel on Exit?"=w383:bool)
        n149 = Select(t="UI: Front Panel State >> Close", s=w383, f="") -> (s? t:f=w380:string)
        n150 = call <vilib>:"Add State(s) to Queue__JKI_lib_State_Machine.vi"("State(s) in (\"\")"=w380, "State(s) at Back (\"\")"="Data: Cleanup\nEvents: Unregister\nExit") -> ("States Out"=w378:string)  [unwired: 13 in]
        n151 = call <vilib>:"Add State(s) to Queue__JKI_lib_State_Machine.vi"("State(s) in Front (\"\")"=w378, "State(s) in (\"\")"=w387) -> ("States Out"=w386:string)  [unwired: 13 in]
      }
      frame "---------- Database ----------" {
        # "Template Separator\n(You can make a copy of, or modify, this frame)"
        n152 = call <vilib>:"Add State(s) to Queue__JKI_lib_State_Machine.vi"("State(s) in (\"\")"=w392) -> ("States Out"=w391:string)  [unwired: 14 in]
      }
      frame "Database: Locate" {
        # "Your code here.\n(You can make a copy of, or modify, this frame)"
        n153 = Unbundle By Name(w398) -> ("SettingDB"=w400:refnum<class "Setting Database.lvclass">)
        n154 = call <vilib>:"Create.vi"("SMO"=refnum<class "SMO.lvclass"> refnum) -> ("error out"=w403:errorcluster, "SMO out"=w405:refnum<class "SMO.lvclass">)  [unwired: 8 in, 1 out]
        n155 = call "Setting Database Name.vi"() -> ("Name"=w401:string)  [unwired: 10 in, 1 out]
        n156 = call <vilib>:"ListSharedResources.vi"("error in (no error)"=w403, "Filter (regex|name)"=w401, "SMO in"=w405) -> ("error out"=w402:errorcluster, "Shared Resources"=w395:refnum<class "SMO.lvclass">[], "SMO out"=w404:refnum<class "SMO.lvclass">)  [unwired: 5 in, 1 out]
        n157 = Index Array(array=w395) -> (element=w396:refnum<class "SMO.lvclass">)  [unwired: 1 in]
        n158 = call <vilib>:"Destroy.vi"("error in (no error)"=w402, "SMO"=w404) -> ()  [unwired: 9 in, 1 out]
        n159 = To More Specific Class(target class=w400, reference=w396) -> (specific class reference=w397:refnum<class "Setting Database.lvclass">)  [unwired: 1 in, 1 out]
        n160 = Bundle By Name(cluster=w398, "SettingDB"=w397) -> (w399:T5)
        n161 = call <vilib>:"Add State(s) to Queue__JKI_lib_State_Machine.vi"("State(s) in (\"\")"=w408) -> ("States Out"=w407:string)  [unwired: 14 in]
      }
      frame "Database: Update Active" {
        # "Your code here.\n(You can make a copy of, or modify, this frame)"
        n162 = Unbundle By Name(w410) -> ("SettingDB"=w416:refnum<class "Setting Database.lvclass">, "Dot Settings"=w415:refnum<class "Dot Settings.lvclass">)
        n163 = call "Setting Database.UpdateActiveDot.vi"("error in (no error)"=w413, "UpdateActiveDot"=w415, "Setting Database"=w416) -> ("error out"=w414:errorcluster, "Setting Database"=w411:refnum<class "Setting Database.lvclass">)  [unwired: 7 in]
        n164 = Bundle By Name(cluster=w410, "SettingDB"=w411) -> (w412:T5)
        n165 = call <vilib>:"Add State(s) to Queue__JKI_lib_State_Machine.vi"("State(s) in (\"\")"=w418) -> ("States Out"=w417:string)  [unwired: 14 in]
      }
    }
  }
